vi "Write panel message Kinetics (SubVI).vi"(4 "rpm":refnum<vi>, 5 "rpm":bool, 6 "PrintTime":bool=TRUE, 7 "Stop":refnum<vi>, 8 "error in (no error)":errorcluster, 9 "Time to wait":dbl, 10 "Strin":string, 11 "String in":refnum<vi>) -> (0 "error out":errorcluster, 1 "RPM":dbl, 2 "Stopped":bool)   [LabVIEW 2017]
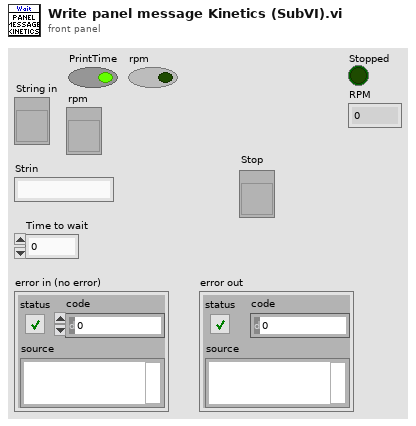
[diagram p1: front panel]
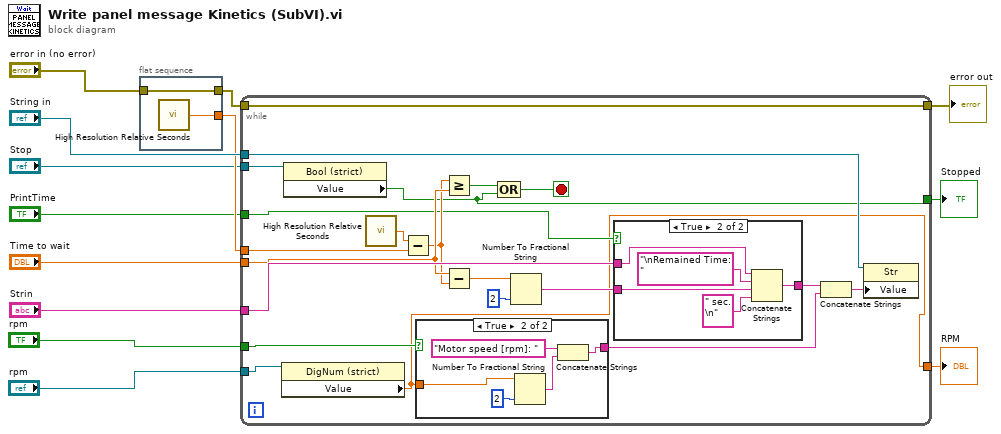
[diagram p0: block diagram]
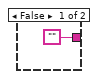
[diagram p2: hidden frame]
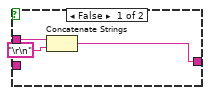
[diagram p3: hidden frame]
diagram:
  n1 = flat-sequence {
    tunnel: [w15] -> w9
    tunnel: "error in (no error)" -> [w15]
    tunnel: [w14] -> w10
    frame #0 {
      n2 = call <vilib>:"High Resolution Relative Seconds.vi"() -> ("relative seconds"=w14:dbl)
    }
  }
  n3 = while {
    tunnel: "Strin" -> [w36]
    tunnel: w9 -> [w31]
    tunnel: w10 -> [w33]
    tunnel: "Time to wait" -> [w27]
    tunnel: [w31] -> w12
    tunnel: "String in" -> [w30]
    tunnel: "Stop" -> [w24]
    tunnel: "PrintTime" -> [w22]
    tunnel: "rpm" -> [w20]
    tunnel: "rpm" -> [w21]
    tunnel: [w17] -> w2
    tunnel: [w16] -> w1
    stop <- w23 stop-if-true
    n4 = property class="DigNum (strict)"(reference=w21) -> ("Value"=w16:dbl)  [unwired: 1 in, 2 out]
    n5 = property class="Bool (strict)"(reference=w24) -> ("Value"=w17:bool)  [unwired: 1 in, 2 out]
    n6 = call <vilib>:"High Resolution Relative Seconds.vi"() -> ("relative seconds"=w34:dbl)
    n7 = Subtract(x=w34, y=w33) -> (x-y=w26:dbl)
    n8 = case shown="True" w20 {
      tunnel: ["" w39] -> w18
      tunnel: w16 -> [_ w38]
      frame False {
      }
      frame True {
        n9 = Number To Fractional String(number=w38, precision (6)=i16 2) -> (F-format string=w40:string)  [unwired: 2 in]
        n10 = Concatenate Strings("Motor speed [rpm]: " ("string"), w40) -> (w39:string)
      }
    }
    n11 = Greater Or Equal?(x=w26, y=w27) -> (x >= y?=w32:bool)
    n12 = Subtract(x=w27, y=w26) -> (x-y=w28:dbl)
    n13 = Compound Arithmetic op=OR(w32, w17) -> (w23:bool)
    n14 = Number To Fractional String(number=w28, precision (6)=i16 2) -> (F-format string=w25:string)  [unwired: 2 in]
    n15 = case shown="True" w22 {
      tunnel: w36 -> [w45 w50]
      tunnel: [w44 w47] -> w35
      tunnel: w25 -> [_ w46]
      frame False {
        n16 = Concatenate Strings(w45, "\r\n") -> (w44:string)
      }
      frame True {
        n17 = Concatenate Strings(w50, "\nRemained Time: " ("string"), w46, " sec.\n" ("string")) -> (w47:string)
      }
    }
    n18 = Concatenate Strings(w35, w18) -> (w19:string)
    n19 = property class="Str"(reference=w30, "Value"=w19) -> ()  [unwired: 1 in, 2 out]
  }
  "error out" <- w12
  "Stopped" <- w2
  "RPM" <- w1
